vi "Multi_Channel_Dynamic_Config.vi"() -> ()   [LabVIEW 2020]
uses:
  <vilib>/Utility/error.llb/DialogType.ctl
  <vilib>/DAQmx/write.llb/DAQmx Write (Analog 1D Wfm NChan NSamp).vi
  <vilib>/DAQmx/create/channels.llb/DAQmx Create Channel (AO-Voltage-Basic).vi
  <vilib>/DAQmx/configure/timing.llb/DAQmx Timing (Sample Clock).vi
  <vilib>/DAQmx/miscellaneous.llb/DAQmx Fill In Error Info.vi
  <resource>/objmgr/daqmx.rc
  <vilib>/measure/NI_MABase.lvlib
panel:
  in  "Phase (Deg)":dbl[](array[numeric])
  in  "Waveform Type":T1(array[ring])
  in  "Desired Frequency":dbl[](array[numeric]) caption="Desired Frequency (Hz)"
  in  "Amplitude":dbl[](array[numeric]) caption="Amplitude (V)"
  in  "Sample Clock Rate":dbl=10000.0 format="%.2f"
  in  "Samples per Buffer":dbl=1000.0
  in  "Physical Channels":tag="Dev1/ao0:1"
  in  "Minimum Value":dbl=-10.0 format="%0.2f"
  in  "Maximum Value":dbl=10.0 format="%0.2f"
  out "Output Data":waveform(dbl)[](graph)=[{"t0"=timestamp(0 s since 1904-01-01), "dt"=2e-05, "Y"=array[250 elements]}]
  in  "stop":bool
  # "DAQmx Task Configuration"
  # "Waveform Attributes"
  # "Introduction: \nThis application demonstrates a method\nfor generating multiple analog waveforms\noutput on multiple channels. It also integrates \na method for dynamically varying the output \nwaveform attributes. All parameters including \nthe waveform type, may be updated at run-\ntime. This example is scalable to any number \nof available channels."
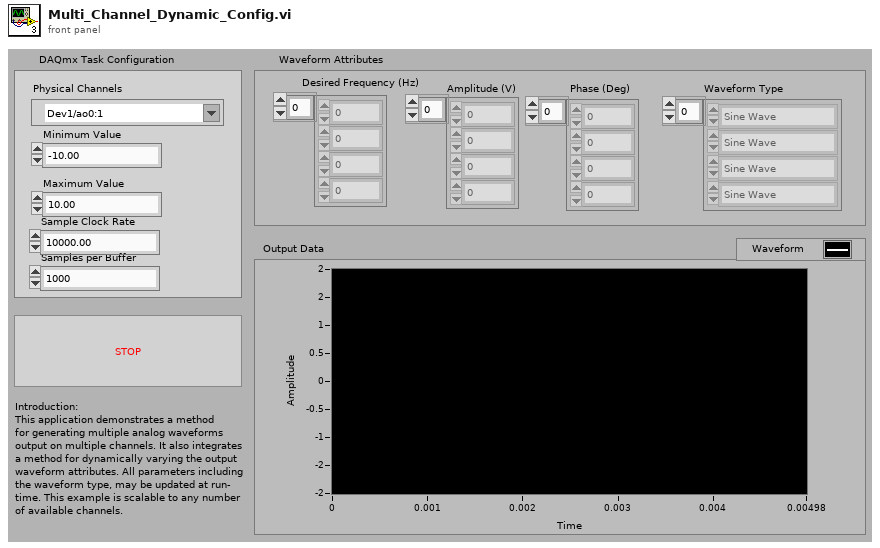
[diagram p1: front panel]
types:
  T1 = enum16{"Sine Wave", "Triangle Wave", "Square Wave", "Sawtooth Wave"}[]
  T2 = typedef "DialogType.ctl" = u16
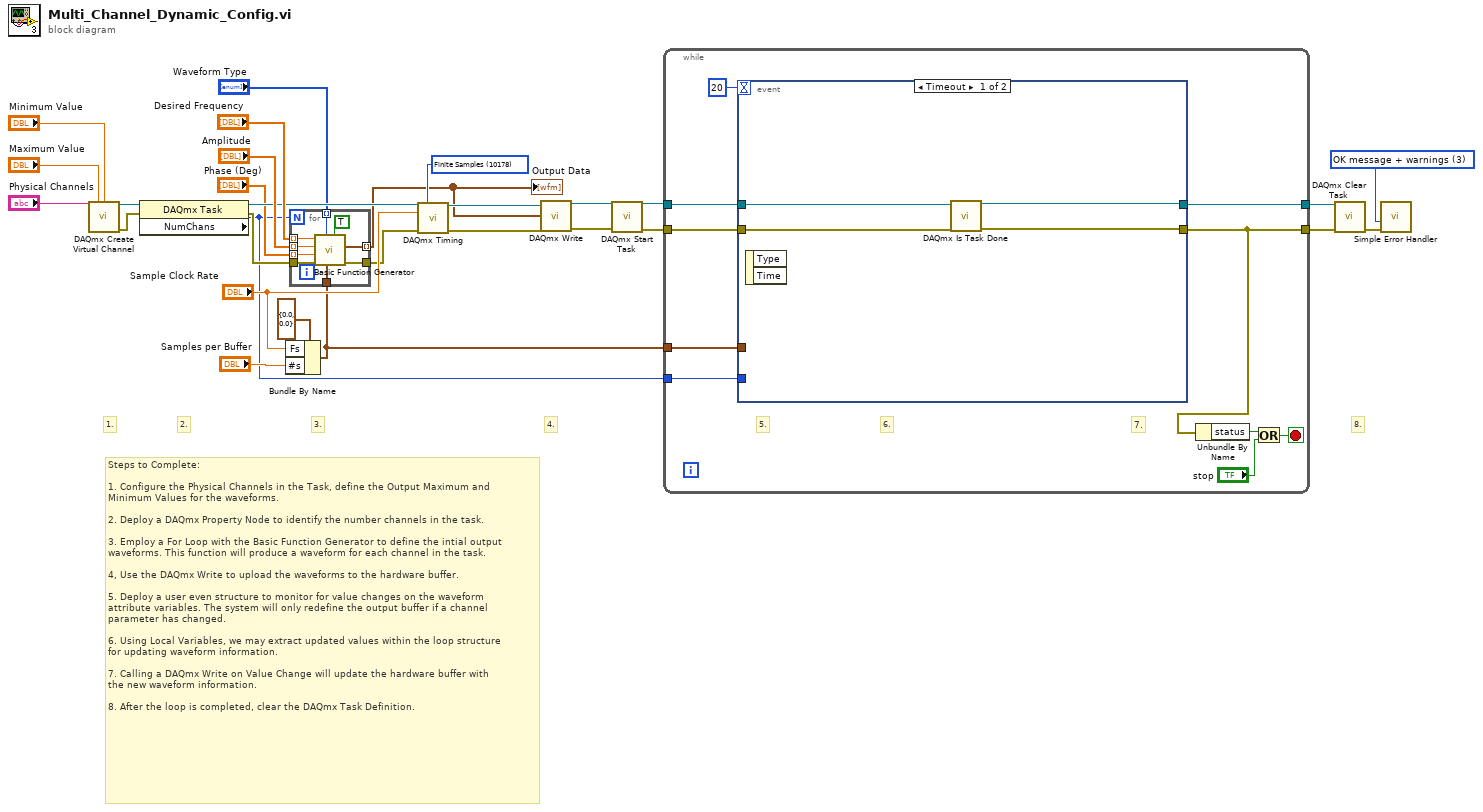
[diagram p0: block diagram]
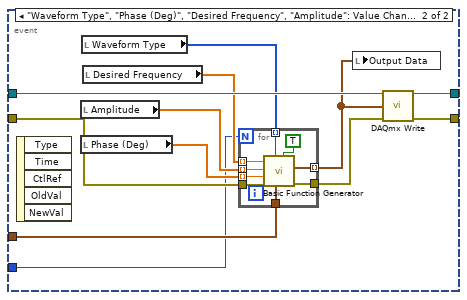
[diagram p2: hidden frame]
diagram:
  w19 = T2 3 items=["no dialog", "OK message", "continue or stop message", "OK message + warnings", "continue/stop + warnings"] ("type of dialog (OK msg:1)")
  w27 = 10178 items=["Finite Samples"=10178, "Continuous Samples"=10123] ("sample mode")
  # "Steps to Complete:\n\n1. Configure the Physical Channels in the Task, define the Output Maximum and \nMinimum Values for the waveforms. \n\n2. Deploy a DAQmx Property Node to identify the number channels in the task. \n\n3. Employ a For Loop with the Basic Function Generator to define the intial output\nwaveforms. This function will produce a waveform for each channel in the task. \n\n4, Use the DAQmx Write to upload the waveforms to the hardware buffer. \n\n5. Deploy a user even structure to monitor for value changes on the waveform \nattribute variables. The system will only redefine the output buffer if a channel \nparameter has changed. \n\n6. Using Local Variables, we may extract updated values within the loop structure\nfor updating waveform information. \n\n7. Calling a DAQmx Write on Value Change will update the hardware buffer with\nthe new waveform information. \n\n8. After the loop is completed, clear the DAQmx Task Definition."
  # "8."
  # "4."
  # "3."
  # "2."
  # "1."
  n1 = call-poly <vilib>:"DAQmx Create Virtual Channel.vi"("maximum value"="Maximum Value", "minimum value"="Minimum Value", "physical channels"="Physical Channels") -> ("task out"=w11:refnum<k21>, "error out"=w7:errorcluster)  [unwired: 11 in]
  n2 = property class="DAQmx Task"(reference=w11, error in=w7) -> (reference out=w10:refnum<k21>, error out=w9:errorcluster, "NumChans"=w3:u32)
  n3 = Bundle By Name(cluster=cluster{"Fs":dbl, "#s":dbl} {"Fs"=0.0, "#s"=0.0} ("sampling info"), "Fs"="Sample Clock Rate", "#s"="Samples per Buffer") -> (w4:cluster{"Fs":dbl, "#s":dbl})
  n4 = for {
    N: w3 -> [_]
    tunnel: w4 -> [w38]
    tunnel: "Amplitude" -> [w37] mode=indexing
    tunnel: "Desired Frequency" -> [w36] mode=indexing
    tunnel: "Waveform Type" -> [w35] mode=indexing
    tunnel: [w34] -> w12
    tunnel: w9 -> [w33]
    tunnel: [w32] -> w8 mode=indexing
    tunnel: "Phase (Deg)" -> [w31] mode=indexing
    n5 = call <vilib>:"Basic Function Generator.vi"("reset signal"=TRUE, "sampling info"=w38, "signal type"=w35, "error in (no error)"=w33, "phase"=w31, "amplitude"=w37, "frequency"=w36) -> ("error out"=w34:errorcluster, "signal out"=w32:waveform(dbl))  [unwired: 2 in, 1 out]
  }
  "Output Data" <- w8
  n6 = call-poly <vilib>:"DAQmx Timing.vi"("task/channels in"=w10, "sample mode"=w27, "rate"="Sample Clock Rate", "error in"=w12) -> ("task out"=w21:refnum<k21>, "error out"=w18:errorcluster)  [unwired: 10 in]
  n7 = call-poly <vilib>:"DAQmx Write.vi"("task/channels in"=w21, "data"=w8, "error in"=w18) -> ("task out"=w24:refnum<k21>, "error out"=w23:errorcluster)  [unwired: 10 in, 1 out]
  n8 = call <vilib>:"DAQmx Start Task.vi"("task/channels in"=w24, "error in"=w23) -> ("task out"=w28:refnum<k21>, "error out"=w22:errorcluster)  [unwired: 12 in]
  n9 = while {
    tunnel: w28 -> [w45]
    tunnel: w22 -> [w44]
    tunnel: w4 -> [w43]
    tunnel: w3 -> [w42]
    tunnel: [w41] -> w2
    tunnel: [w40] -> w1
    stop <- w47 stop-if-true
    # "7."
    # "6."
    # "5."
    n10 = event shown="[0] Timeout" {
      selector: _ -> [_ _]
      dyn-events: _ -> [_ _]
      timeout: 20 -> [_ _]
      tunnel: w45 -> [w52 w64]
      tunnel: w44 -> [w51 w63]
      tunnel: w43 -> [_ w57]
      tunnel: [w50 w56] -> w41
      tunnel: [w49 w55] -> w40
      tunnel: w42 -> [_ w53]
      event Timeout {
        n11 = event-data() -> ()  [unwired: 1 in, 2 out]
        n12 = call <vilib>:"DAQmx Is Task Done.vi"("task/channels in"=w52, "error in"=w51) -> ("task out"=w50:refnum<k21>, "error out"=w49:errorcluster)  [unwired: 11 in, 1 out]
      }
      event "Waveform Type", "Phase (Deg)", "Desired Frequency", "Amplitude": Value Change {
        n13 = event-data() -> ()  [unwired: 1 in, 5 out]
        n14 = local read "Amplitude"() -> (w60:dbl[])
        n15 = local read "Phase (Deg)"() -> (w59:dbl[])
        n16 = local read "Waveform Type"() -> (w58:T1)
        n17 = local read "Desired Frequency"() -> (w61:dbl[])
        n18 = for {
          N: w53 -> [_]
          tunnel: [w73] -> w62
          tunnel: [w72] -> w54 mode=indexing
          tunnel: w63 -> [w71]
          tunnel: w61 -> [w70] mode=indexing
          tunnel: w60 -> [w69] mode=indexing
          tunnel: w59 -> [w68] mode=indexing
          tunnel: w58 -> [w66] mode=indexing
          tunnel: w57 -> [w65]
          n19 = call <vilib>:"Basic Function Generator.vi"("reset signal"=TRUE, "sampling info"=w65, "signal type"=w66, "error in (no error)"=w71, "phase"=w68, "amplitude"=w69, "frequency"=w70) -> ("error out"=w73:errorcluster, "signal out"=w72:waveform(dbl))  [unwired: 2 in, 1 out]
        }
        n20 = local write "Output Data"(w54) -> ()
        n21 = call-poly <vilib>:"DAQmx Write.vi"("task/channels in"=w64, "data"=w54, "error in"=w62) -> ("task out"=w56:refnum<k21>, "error out"=w55:errorcluster)  [unwired: 10 in, 1 out]
      }
    }
    n22 = Unbundle By Name(w40) -> ("status"=w39:bool)
    n23 = Or(x=w39, y="stop") -> (x .or. y?=w47:bool)
  }
  n24 = call <vilib>:"DAQmx Clear Task.vi"("task in"=w2, "error in"=w1) -> ("error out"=w29:errorcluster)  [unwired: 13 in]
  n25 = call <vilib>:"Simple Error Handler.vi"("type of dialog (OK msg:1)"=w19, "error in (no error)"=w29) -> ()  [unwired: 3 in, 5 out]
